vi "Get Data from two FIFOs.vi"(5 "FIFO1":refnum<k21>="FIFOtoFFTLoop", 7 "FIFO0":refnum<k21>="FIFOtoFFTLoop", 8 "Get New Data":bool, 9 "Current Input Index":u16, 11 "FFT State Info":T1) -> (0 "Data Valid":bool, 1 "FXP Data":fxp<+/-,16,2>, 2 "Data":i16, 3 "FFT State Info Out":T1)   [LabVIEW 2012]
uses:
  <vilib>/rvi/DataTransferAndStorage/Container/Common/niFpgaContainerExecOnDevCompGetState.vi
  <vilib>/rvi/Emulation/niFpgaSctlEmulationGetInTimedLoop.vi
  <vilib>/rvi/DataTransferAndStorage/Container/Common/niFpgaContainerGetUniqueNameForEmu.vi
  <vilib>/rvi/FIFO/Fifo_Resource/nirvififoEmulationSetSize.vi
  <vilib>/rvi/Emulation/niFpgaSctlEmulationFifoFullMgr.vi
  <vilib>/rvi/errors/niFpgaSetErrorForExecOnDevCompSimple.vi
  <vilib>/rvi/eio/common/nirviEmuReportErrorAndStop.vi
  <vilib>/rvi/interface/RandomDataEmulation/nirviRandomDataFPGAFIFO.vi
  <vilib>/rvi/interface/RandomDataEmulation/niFpgaRandomDataHandleErrors.vi
  <vilib>/rvi/FXPMathLib/basic elements/FxpDiscreteDelay/XNode/nifxpmath_DiscreteDelay.xnode
  <vilib>/rvi/DataTransferAndStorage/Container/XNode/niFpgaContainer.xnode
  <vilib>/rvi/FIFO/Fifo_Resource/niFpgaFifoEmulationRefIn.vi
  <vilib>/rvi/FXPMathLib/FxpInterpret/XNode/nifxpmath_Interpret.xnode
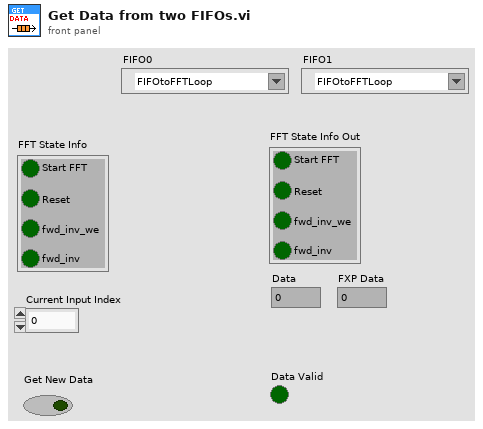
[diagram p1: front panel]
types:
  T1 = cluster{"Reset":bool, "Start FFT":bool, "fwd_inv_we":bool, "fwd_inv":bool}
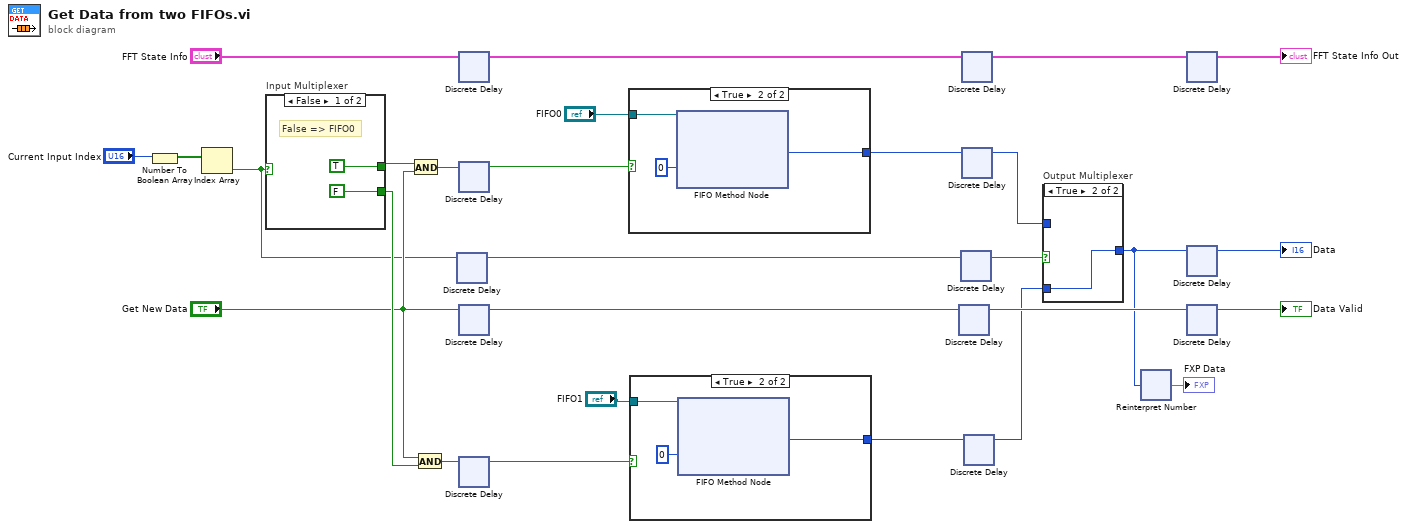
[diagram p0: block diagram]
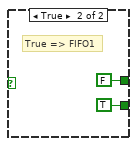
[diagram p3: hidden frame]
diagram:
  n1 = Number To Boolean Array(number="Current Input Index") -> (Boolean array=w11:bool[])
  n2 = Index Array(array=w11) -> (element=w8:bool)  [unwired: 1 in]
  n3 = case "Input Multiplexer" shown="False" w8 {
    tunnel: [TRUE FALSE] -> w17
    tunnel: [FALSE TRUE] -> w15
    frame False {
      # "False => FIFO0"
    }
    frame True {
      # "True => FIFO1"
    }
  }
  n4 = And(x=w17, y="Get New Data") -> (x .and. y?=w16:bool)
  n5 = And(x="Get New Data", y=w15) -> (x .and. y?=w14:bool)
  n6 = xnode "Discrete Delay"("D"=w8) -> ("Q"=w7:bool)
  n7 = xnode "Discrete Delay"("D"="FFT State Info") -> ("Q"=w27:T1)
  n8 = xnode "Discrete Delay"("D"=w16) -> ("Q"=w20:bool)
  n9 = xnode "Discrete Delay"("D"="Get New Data") -> ("Q"=w18:bool)
  n10 = xnode "Discrete Delay"("D"=w14) -> ("Q"=w19:bool)
  n11 = case shown="True" w20 {
    tunnel: [_ w33] -> w26
    tunnel: "FIFO0" -> [_ w35]
    frame False {
    }
    frame True {
      n12 = xnode ("FIFO Method Node")("Timeout"=0, "FIFO In"=w35) -> ("Element"=w33:i16)  [unwired: 2 out]
    }
  }
  n13 = case shown="True" w19 {
    tunnel: [_ w37] -> w21
    tunnel: "FIFO1" -> [_ w36]
    frame False {
    }
    frame True {
      n14 = xnode ("FIFO Method Node")("Timeout"=0, "FIFO In"=w36) -> ("Element"=w37:i16)  [unwired: 2 out]
    }
  }
  n15 = xnode "Discrete Delay"("D"=w18) -> ("Q"=w23:bool)
  n16 = xnode "Discrete Delay"("D"=w7) -> ("Q"=w6:bool)
  n17 = xnode "Discrete Delay"("D"=w27) -> ("Q"=w25:T1)
  n18 = xnode "Discrete Delay"("D"=w26) -> ("Q"=w10:i16)
  n19 = xnode "Discrete Delay"("D"=w21) -> ("Q"=w9:i16)
  n20 = case "Output Multiplexer" shown="True" w6 {
    tunnel: w10 -> [w39 _]
    tunnel: w9 -> [_ w40]
    tunnel: [w39 w40] -> w2
    frame False {
    }
    frame True {
    }
  }
  n21 = xnode "Reinterpret Number"("x"=w2) -> ("y"=→"FXP Data":fxp<+/-,16,2>)
  n22 = xnode "Discrete Delay"("D"=w25) -> ("Q"=→"FFT State Info Out":T1)
  n23 = xnode "Discrete Delay"("D"=w2) -> ("Q"=→"Data":i16)
  n24 = xnode "Discrete Delay"("D"=w23) -> ("Q"=→"Data Valid":bool)
